vi "Begin.vi"() -> (0 "error out":errorcluster)   [LabVIEW 2013]
doc: "Called before other user functions, this VI is expected to open initial I/O refnums, load in file data, and do all program initialization. Notice that the <B>error out</B> terminal is simply used for data flow. Wiring it to other structures or subVIs ensures that this VI runs first."
uses:
  <vilib>/Rock Robotics/WPI/Camera/WPI_CameraImageSize.ctl
  <vilib>/Rock Robotics/SystemInterfaces/DIO/FPGA_DIOPWMChannel.ctl
  <vilib>/Rock Robotics/WPI/DriverStation/WPI_DriverStationRobotMode2.ctl
  <vilib>/Rock Robotics/WPI/Joystick/WPI_JoystickDeviceEnum.ctl
  <vilib>/Rock Robotics/SystemInterfaces/DIO/FPGA_DIOChannel.ctl
  <vilib>/Rock Robotics/WPI/Camera/WPI_CameraWhite Balance Values.ctl
  <vilib>/Rock Robotics/WPI/Camera/WPI_CameraExposure Values.ctl
  <vilib>/Rock Robotics/WPI/Camera/WPI_CameraFrameRate.ctl
  <vilib>/Rock Robotics/SystemInterfaces/Typedef/FPGA_TypedefSolenoidModule.ctl
  <vilib>/Rock Robotics/WPI/Solenoid/WPI_SolenoidChannel.ctl
  <vilib>/Rock Robotics/SystemInterfaces/Typedef/FPGA_TypedefDigitalModule.ctl
  <vilib>/Rock Robotics/SystemInterfaces/DIO/FPGA_DIORelayChannel.ctl
  <vilib>/Rock Robotics/SystemInterfaces/Typedef/FPGA_TypedefAnalogModule.ctl
  <vilib>/Rock Robotics/SystemInterfaces/AI/FPGA_AIChannel.ctl
  <vilib>/Rock Robotics/WPI/Encoder/WPI_EncoderType.ctl
  <vilib>/Rock Robotics/WPI/Relay/WPI_RelayDirection.ctl
  <vilib>/Rock Robotics/WPI/RobotDrive/WPI_RobotDriveOpen2MotorWithTalon.vi
  Robot Global Data.vi
  <vilib>/Rock Robotics/WPI/MotorControl/WPI_MotorControlOpen Talon.vi
  <vilib>/Rock Robotics/WPI/Counter/WPI_CounterDigitalInputToDigitalSource.vi
  <vilib>/Rock Robotics/WPI/Solenoid/WPI_SolenoidOpenDouble.vi
  <vilib>/Rock Robotics/WPI/Compressor/WPI_CompressorGetSetRefNum.vi
panel:
  in  "Image Size 2":T1=enum."160x120"
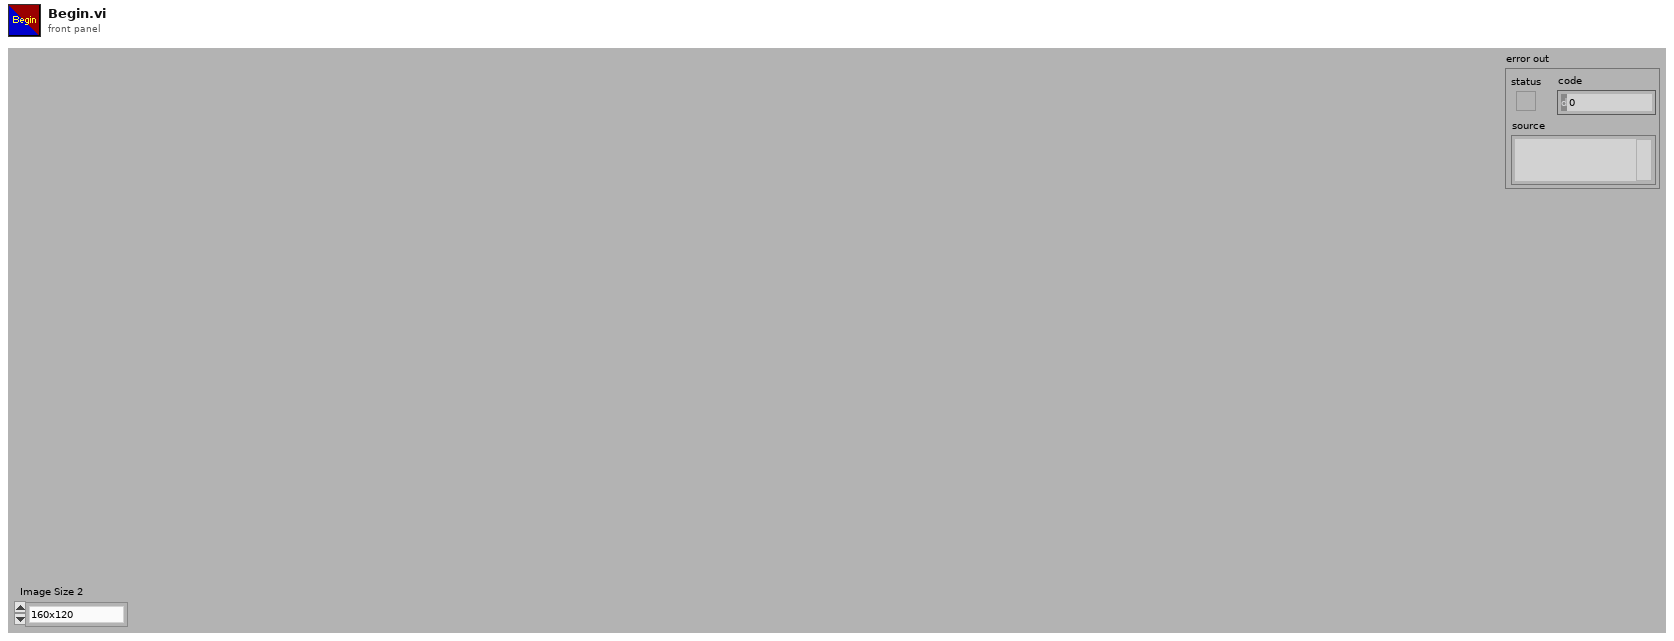
[diagram p1: front panel]
types:
  T1 = typedef "WPI_CameraImageSize.ctl" = enum16{"640x480", "320x240", "160x120"}
  T2 = typedef "WPI_JoystickDeviceEnum.ctl" = enum16{"USB 1", "USB 2", "USB 3", "USB 4", "Kinect 1", "Kinect 2"}
  T3 = typedef "WPI_RelayDirection.ctl" = enum16{"Both directions", "Forward only", "Reverse only"}
  T4 = typedef "FPGA_DIORelayChannel.ctl" = enum8{"Relay 1", "Relay 2", "Relay 3", "Relay 4", "Relay 5", "Relay 6", "Relay 7", "Relay 8", "Invalid"}
  T5 = typedef "FPGA_TypedefDigitalModule.ctl" = enum16{"Digital Module 1", "Digital Module 2"}
  T6 = typedef "FPGA_DIOChannel.ctl" = enum8{"DIO 1", "DIO 2", "DIO 3", "DIO 4", "DIO 5", "DIO 6", "DIO 7", "DIO 8", "DIO 9", "DIO 10", "DIO 11", "DIO 12", "DIO 13", "DIO 14", "Invalid"}
  T7 = typedef "WPI_EncoderType.ctl" = enum16{"1x", "2x", "4x"}
  T8 = typedef "FPGA_AIChannel.ctl" = enum8{"AI 1", "AI 2", "AI 3", "AI 4", "AI 5", "AI 6", "AI 7", "AI 8", "Invalid"}
  T9 = typedef "FPGA_TypedefAnalogModule.ctl" = enum16{"Analog Module 1", "Analog Module 2"}
  T10 = typedef "WPI_SolenoidChannel.ctl" = enum8{"Solenoid 1", "Solenoid 2", "Solenoid 3", "Solenoid 4", "Solenoid 5", "Solenoid 6", "Solenoid 7", "Solenoid 8", "Invalid"}
  T11 = typedef "FPGA_TypedefSolenoidModule.ctl" = enum16{"Solenoid Module 1", "Solenoid Module 2"}
  T12 = typedef "FPGA_DIOPWMChannel.ctl" = enum8{"PWM 1", "PWM 2", "PWM 3", "PWM 4", "PWM 5", "PWM 6", "PWM 7", "PWM 8", "PWM 9", "PWM 10", "Invalid"}
  T13 = typedef "WPI_CameraFrameRate.ctl" = u32
  T14 = typedef "WPI_CameraExposure Values.ctl" = enum16{"Auto", "Flicker-free 50 Hz", "Flicker-free 60 Hz", "Hold current"}
  T15 = typedef "WPI_CameraWhite Balance Values.ctl" = enum16{"Auto", "Fixed indoor", "Fixed outdoor 1", "Fixed outdoor 2", "Fixed fluorescent 1", "Fixed fluorescent 2", "Hold current"}
  T16 = typedef "WPI_DriverStationRobotMode2.ctl" = enum16{"Autonomous Disabled", "Autonomous Enabled", "Teleop Disabled", "Teleop Enabled", "Timeout", "Finish", "Test Disabled", "Test Enabled"}
  T17 = typedef "WPI_DigitalInputDevRef.ctl" = cluster{"DevStatus":errorcluster, "DIO Channel":T6, "Digital Module":T5}
  T18 = typedef "FPGA_CounterEncoderSourceConvertionLVSourceType.ctl" = cluster{"DevStatus":errorcluster, "AnalogTriggerMode?":bool, "DigitalMode":cluster{"Digital Module":T5, "DIO Channel":T19}, "AnalogTriggerMode":cluster{"AnalogTriggerIndex":T20, "OutputType":T21}}
  T19 = typedef "FPGA_DIODigitalSourceChannel.ctl" = enum8{"DIO 1", "DIO 2", "DIO 3", "DIO 4", "DIO 5", "DIO 6", "DIO 7", "DIO 8", "DIO 9", "DIO 10", "DIO 11", "DIO 12", "DIO 13", "DIO 14", "Disabled"}
  T20 = typedef "FPGA_AnalogTriggerIndex.ctl" = enum8{"Trig 0", "Trig 1", "Trig 2", "Trig 3", "Trig 4", "Trig 5", "Trig 6", "Trig 7", "Invalid"}
  T21 = typedef "FPGA_AnalogTriggerOutType.ctl" = enum16{"InWindow", "TriggerState", "Rising", "Falling"}
  T22 = typedef "WPI_EncoderDevRef.ctl" = cluster{"DevStatus":errorcluster, "EncoderIndex":T23, "CounterIndex":T24, "DistancePerCount":dbl, "Decoding Type":T7}
  T23 = typedef "FPGA_EncoderIdx.ctl" = enum8{"Enc 0", "Enc 1", "Enc 2", "Enc 3", "Invalid"}
  T24 = typedef "FPGA_CounterCtrSystemIndex.ctl" = enum8{"Ctr 0", "Ctr 1", "Ctr 2", "Ctr 3", "Ctr 4", "Ctr 5", "Ctr 6", "Ctr 7", "Invalid"}
  T25 = typedef "WPI_JoystickDevRef.ctl" = cluster{"Device":T2}
  T26 = typedef "WPI_CompressorDevRef.ctl" = cluster{"DevStatus":errorcluster, "DigitalInputDevRef":T17, "RelayDevRef":T27}
  T27 = typedef "WPI_RelayDevRef.ctl" = cluster{"DevStatus":errorcluster, "Relay Channel":T4, "Digital Module":T5, "Relay Direction":T3}
  T28 = typedef "WPI_RobotDriveDevRef.ctl" = cluster{"DevStatus":errorcluster, "Motors[]":T29[], "Square Inputs":bool, "Max Output":dbl, "Isochronous":bool}
  T29 = typedef "WPI_MotorControlDeviceRef.ctl" = cluster{"DeviceStatus":errorcluster, "Type":enum16{"PWM", "CAN"}, "PWM":cluster{"Digital Module":T5, "PWM Channel":T12, "DeadBand":T30}, "CAN":cluster{"Device Number":u8, "Control Mode":T31, "Semaphore":T32, "Max Vout":dbl}, "Invert":bool, "TransformRef":T33, "InvTransformRef":T33}
  T30 = typedef "WPI_PWMDeadband.ctl" = cluster{"Name":string, "maxPositivePwm":i32, "minPositivePwm":i32, "centerPwm":i32, "maxNegativePwm":i32, "minNegativePwm":i32, "angularRange":u16}
  T31 = typedef "WPI_CANJaguar_ControlMode.ctl" = enum8{"Percent VBus", "Current", "Speed", "Position", "Voltage"}
  T32 = typedef "Semaphore RefNum" = refnum<k1>
  T33 = typedef "WPI_PWMTransform_ConPane.ctl" = refnum<vi>
  T34 = typedef "WPI_SolenoidDevRef.ctl" = cluster{"DevStatus":errorcluster, "Solenoid Module":T11, "Forward Solenoid Channel":T10, "Reverse Solenoid Channel":T10}
  T35 = typedef "WPI_CameraDevRef.ctl" = cluster{"Camera Address":string, "CameraStatus":errorcluster, "Acquire Image Notifier":refnum<notifier>}
  T36 = typedef "WPI_ServoDeviceRef.ctl" = cluster{"DeviceStatus":errorcluster, "Digital Module":T5, "PWM Channel":T12, "DeadBand":T30}
  T37 = typedef "WPI_AnalogChannelDevRef.ctl" = cluster{"DevStatus":errorcluster, "Analog Module":T9, "Analog Channel":T8}
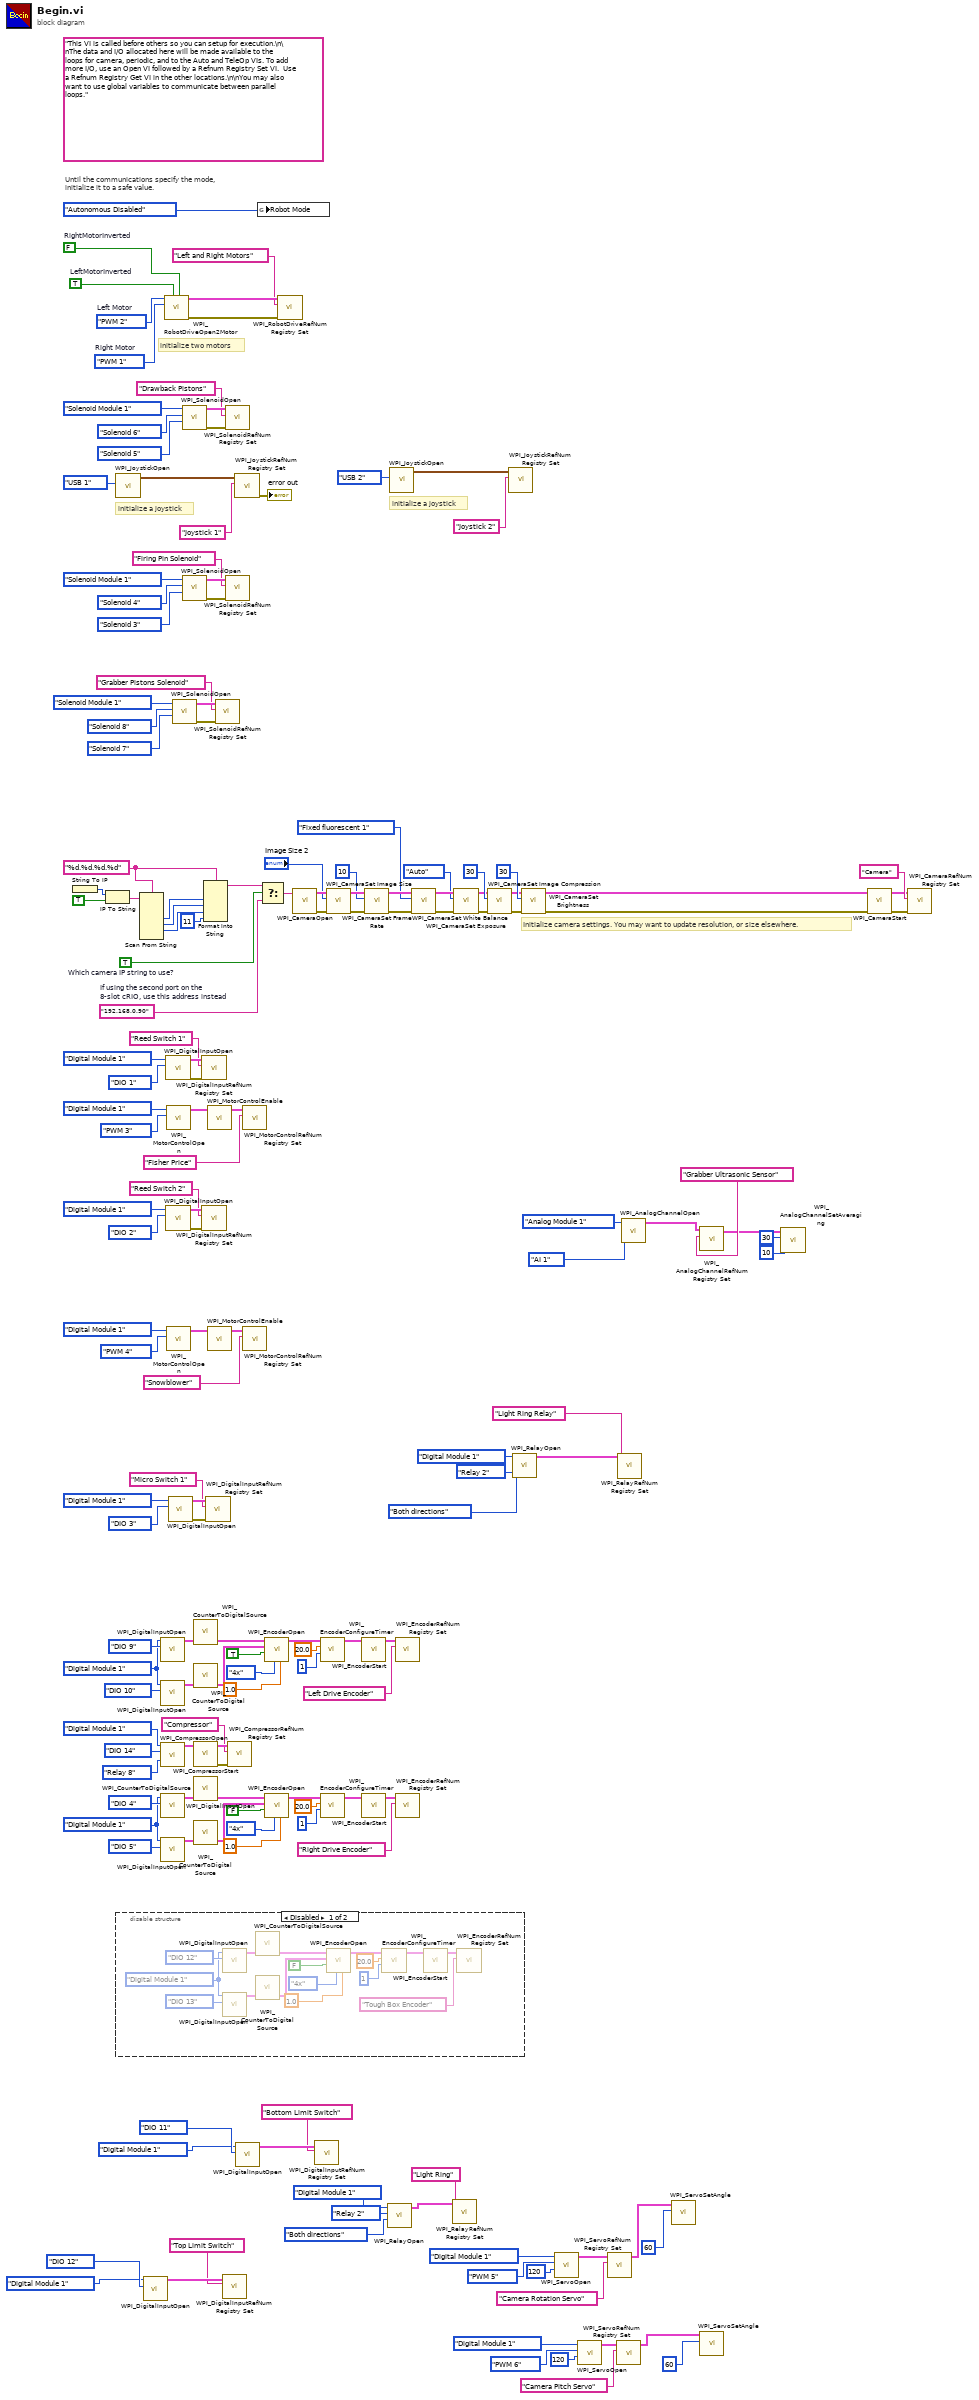
[diagram p0: block diagram]
diagram:
  w25 = FPGA_TypedefDigitalModule."Digital Module 1" ("DIO Module")
  w108 = TRUE  # Which camera IP string to use?
  w112 = "%d.%d.%d.%d" ("format string")
  w109 = "192.168.0.90"  # If using the second port on the 8-slot cRIO, use this address instead
  w141 = FPGA_TypedefDigitalModule."Digital Module 1" ("DIO Module")
  (unwired) "This VI is called before others so you can setup for execution.\n\nThe data and I/O allocated here will be made available to the loops for camera, periodic, and to the Auto and TeleOp VIs. To add more I/O, use an Open VI followed by a Refnum Registry Set VI.  Use a Refnum Registry Get VI in the other locations.\n\nYou may also want to use global variables to communicate between parallel loops."
  w165 = FPGA_DIOPWMChannel."PWM 1"  # Right Motor
  w166 = FPGA_DIOPWMChannel."PWM 2"  # Left Motor
  w170 = TRUE  # LeftMotorInverted
  w171 = FALSE  # RightMotorInverted
  # "initialize a joystick"
  # "Initialize camera settings. You may want to update resolution, or size elsewhere."
  # "initialize a joystick"
  # "Until the communications specify the mode,\ninitialize it to a safe value."
  # "initialize two motors"
  n1 = String To IP() -> (0:w119:u32)  [unwired: 1 in]
  n2 = IP To String(1:TRUE ("dot notation? (F)"), 2:w119) -> (0:w117:string)
  n3 = disable-structure shown="Disabled" {
    frame Disabled {
      w174 = FPGA_TypedefDigitalModule."Digital Module 1" ("DIO Module")
      n4 = call <vilib>:"WPI_DigitalInputOpen.vi"("DIO Channel"=FPGA_DIOChannel."DIO 12" ("A Channel"), "Digital Module (Module 1)"=w174) -> ("DigitalInputDevRef"=w185:T17)  [unwired: 1 in, 8 out]
      n5 = call <vilib>:"WPI_DigitalInputOpen.vi"("DIO Channel"=FPGA_DIOChannel."DIO 13" ("B Channel"), "Digital Module (Module 1)"=w174) -> ("DigitalInputDevRef"=w186:T17)  [unwired: 1 in, 8 out]
      n6 = call-poly <vilib>:"WPI_CounterToDigitalSource.vi"("DigitalInputDevRef"=w185) -> ("Digital Source"=w184:T18)  [unwired: 6 out]
      n7 = call-poly <vilib>:"WPI_CounterToDigitalSource.vi"("DigitalInputDevRef"=w186) -> ("Digital Source"=w187:T18)  [unwired: 6 out]
      n8 = call <vilib>:"WPI_EncoderOpen.vi"("DistancePerCount"=1.0, "Decoding Type"=WPI_EncoderType."4x", "Invert Direction (False)"=FALSE ("Invert Direction"), "BSource"=w187, "ASource"=w184) -> ("EncoderDevRef"=w177:T22)  [unwired: 3 in, 3 out]
      n9 = call <vilib>:"WPI_EncoderConfigureTimer.vi"("Number Samples to Average"=u8 1, "Minimum Rate"=20.0, "EncoderDevRef"=w177) -> ("EncoderDevRef"=w178:T22)  [unwired: 1 in, 7 out]
      n10 = call <vilib>:"WPI_EncoderStart.vi"("EncoderDevRef"=w178) -> ("EncoderDevRef"=w173:T22)  [unwired: 1 in, 9 out]
      n11 = call <vilib>:"WPI_EncoderRefNum Registry Set.vi"("refnum name"="Tough Box Encoder", "EncoderDevRef"=w173) -> ()  [unwired: 8 in, 2 out]
    }
    frame Enabled {
    }
  }
  n12 = call <vilib>:"WPI_JoystickOpen.vi"("JoystickDevice"=WPI_JoystickDeviceEnum."USB 1") -> ("JoystickDevRef"=w162:T25)  [unwired: 10 in]
  n13 = Scan From String(format string=w112, input string=w117) -> (output 1=w116:i32, output 2=w115:i32, output 3=w114:i32)  [unwired: 7 in, 3 out]
  n14 = call <vilib>:"WPI_DigitalInputOpen.vi"("DIO Channel"=FPGA_DIOChannel."DIO 12" ("A Channel"), "Digital Module (Module 1)"=FPGA_TypedefDigitalModule."Digital Module 1" ("DIO Module")) -> ("DigitalInputDevRef"=w40:T17)  [unwired: 8 in, 1 out]
  n15 = call <vilib>:"WPI_DigitalInputOpen.vi"("DIO Channel"=FPGA_DIOChannel."DIO 9" ("A Channel"), "Digital Module (Module 1)"=w25) -> ("DigitalInputDevRef"=w36:T17)  [unwired: 1 in, 8 out]
  n16 = call <vilib>:"WPI_DigitalInputOpen.vi"("DIO Channel"=FPGA_DIOChannel."DIO 10" ("B Channel"), "Digital Module (Module 1)"=w25) -> ("DigitalInputDevRef"=w37:T17)  [unwired: 1 in, 8 out]
  n17 = call <vilib>:"WPI_CompressorOpen.vi"("Pressure Switch Digital Module (Module 1)"=FPGA_TypedefDigitalModule."Digital Module 1" ("Switch and Relay Module"), "Pressure Switch DIO Channel"=FPGA_DIOChannel."DIO 14" ("Pressure Switch Channel"), "Relay Channel"=FPGA_DIORelayChannel."Relay 8" ("RelayChannel")) -> ("CompressorDevRef"=w96:T26)  [unwired: 2 in, 10 out]
  n18 = call <vilib>:"WPI_DigitalInputOpen.vi"("DIO Channel"=FPGA_DIOChannel."DIO 4" ("A Channel"), "Digital Module (Module 1)"=w141) -> ("DigitalInputDevRef"=w152:T17)  [unwired: 1 in, 8 out]
  n19 = call <vilib>:"WPI_DigitalInputOpen.vi"("DIO Channel"=FPGA_DIOChannel."DIO 5" ("B Channel"), "Digital Module (Module 1)"=w141) -> ("DigitalInputDevRef"=w153:T17)  [unwired: 1 in, 8 out]
  n20 = call-poly <vilib>:"WPI_RobotDriveOpen2Motor.vi"("Right Motor Inverted"=w171, "Left Motor Inverted"=w170, "Right Motor"=w165, "Left Motor"=w166) -> ("error out"=w167:errorcluster, "RobotDriveDevRef"=w169:T28)  [unwired: 1 in, 5 out]
  n21 = call <vilib>:"WPI_DigitalInputOpen.vi"("DIO Channel"=FPGA_DIOChannel."DIO 1" ("Limit Switch Channel"), "Digital Module (Module 1)"=FPGA_TypedefDigitalModule."Digital Module 1" ("Switch and Relay Module")) -> ("error out"=w95:errorcluster, "DigitalInputDevRef"=w94:T17)  [unwired: 1 in, 7 out]
  n22 = call <vilib>:"WPI_DigitalInputOpen.vi"("DIO Channel"=FPGA_DIOChannel."DIO 2" ("Limit Switch Channel"), "Digital Module (Module 1)"=FPGA_TypedefDigitalModule."Digital Module 1" ("Switch and Relay Module")) -> ("error out"=w77:errorcluster, "DigitalInputDevRef"=w76:T17)  [unwired: 1 in, 7 out]
  n23 = call-poly <vilib>:"WPI_MotorControlOpen.vi"("PWM Channel"=FPGA_DIOPWMChannel."PWM 3" ("Left Motor"), "Digital Module (Module 1)"=enum16{"Digital Module 1"}."Digital Module 1") -> ("MotorControlDeviceRef"=w73:T29)  [unwired: 8 in, 1 out]
  n24 = call-poly <vilib>:"WPI_MotorControlOpen.vi"("PWM Channel"=FPGA_DIOPWMChannel."PWM 4" ("Left Motor"), "Digital Module (Module 1)"=enum16{"Digital Module 1"}."Digital Module 1") -> ("MotorControlDeviceRef"=w71:T29)  [unwired: 8 in, 1 out]
  n25 = call <vilib>:"WPI_DigitalInputOpen.vi"("DIO Channel"=FPGA_DIOChannel."DIO 3", "Digital Module (Module 1)"=FPGA_TypedefDigitalModule."Digital Module 1") -> ("error out"=w19:errorcluster, "DigitalInputDevRef"=w20:T17)  [unwired: 1 in, 7 out]
  n26 = call-poly <vilib>:"WPI_SolenoidOpen.vi"("Reverse Solenoid Channel"=WPI_SolenoidChannel."Solenoid 7" ("Extend Solenoid Channel"), "Forward Solenoid Channel"=WPI_SolenoidChannel."Solenoid 8" ("Retract Solenoid Channel"), "Solenoid Module (Module 1)"=FPGA_TypedefSolenoidModule."Solenoid Module 1" ("Solenoid Module")) -> ("error out"=w52:errorcluster, "SolenoidDevRef"=w51:T34)  [unwired: 1 in, 6 out]
  n27 = call-poly <vilib>:"WPI_SolenoidOpen.vi"("Reverse Solenoid Channel"=WPI_SolenoidChannel."Solenoid 5" ("Extend Solenoid Channel"), "Forward Solenoid Channel"=WPI_SolenoidChannel."Solenoid 6" ("Retract Solenoid Channel"), "Solenoid Module (Module 1)"=FPGA_TypedefSolenoidModule."Solenoid Module 1" ("Solenoid Module")) -> ("error out"=w92:errorcluster, "SolenoidDevRef"=w91:T34)  [unwired: 1 in, 6 out]
  n28 = call-poly <vilib>:"WPI_SolenoidOpen.vi"("Reverse Solenoid Channel"=WPI_SolenoidChannel."Solenoid 3" ("Extend Solenoid Channel"), "Forward Solenoid Channel"=WPI_SolenoidChannel."Solenoid 4" ("Retract Solenoid Channel"), "Solenoid Module (Module 1)"=FPGA_TypedefSolenoidModule."Solenoid Module 1" ("Solenoid Module")) -> ("error out"=w83:errorcluster, "SolenoidDevRef"=w82:T34)  [unwired: 1 in, 6 out]
  n29 = call-poly <vilib>:"WPI_CounterToDigitalSource.vi"("DigitalInputDevRef"=w36) -> ("Digital Source"=w35:T18)  [unwired: 6 out]
  n30 = call-poly <vilib>:"WPI_CounterToDigitalSource.vi"("DigitalInputDevRef"=w37) -> ("Digital Source"=w38:T18)  [unwired: 6 out]
  n31 = call <vilib>:"WPI_CompressorStart.vi"("CompressorDevRef"=w96) -> ("error out"=w89:errorcluster, "CompressorDevRef"=w88:T26)  [unwired: 1 in, 8 out]
  n32 = call-poly <vilib>:"WPI_CounterToDigitalSource.vi"("DigitalInputDevRef"=w152) -> ("Digital Source"=w151:T18)  [unwired: 6 out]
  n33 = call-poly <vilib>:"WPI_CounterToDigitalSource.vi"("DigitalInputDevRef"=w153) -> ("Digital Source"=w154:T18)  [unwired: 6 out]
  n34 = call <vilib>:"WPI_DigitalInputRefNum Registry Set.vi"("error in (no error)"=w95, "refnum name"="Reed Switch 1", "DigitalInputDevRef"=w94) -> ()  [unwired: 7 in, 2 out]
  n35 = call <vilib>:"WPI_DigitalInputRefNum Registry Set.vi"("error in (no error)"=w77, "refnum name"="Reed Switch 2", "DigitalInputDevRef"=w76) -> ()  [unwired: 7 in, 2 out]
  n36 = Format Into String(format string=w112, w116, w115, w114, 11 ("Compression")) -> (resulting string=w110:string)  [unwired: 2 in, 1 out]
  n37 = call <vilib>:"WPI_DigitalInputRefNum Registry Set.vi"("error in (no error)"=w19, "refnum name"="Micro Switch 1", "DigitalInputDevRef"=w20) -> ()  [unwired: 7 in, 2 out]
  n38 = call <vilib>:"WPI_MotorControlEnable.vi"("CAN Jaguar Ref"=w73) -> ("CAN Jaguar Ref Out"=w72:T29)  [unwired: 9 in, 1 out]
  n39 = call <vilib>:"WPI_MotorControlEnable.vi"("CAN Jaguar Ref"=w71) -> ("CAN Jaguar Ref Out"=w70:T29)  [unwired: 9 in, 1 out]
  n40 = call <vilib>:"WPI_SolenoidRefNum Registry Set.vi"("error in (no error)"=w52, "refnum name"="Grabber Pistons Solenoid", "SolenoidDevRef"=w51) -> ()  [unwired: 7 in, 2 out]
  n41 = call <vilib>:"WPI_DigitalInputRefNum Registry Set.vi"("refnum name"="Top Limit Switch", "DigitalInputDevRef"=w40) -> ()  [unwired: 8 in, 2 out]
  n42 = call <vilib>:"WPI_SolenoidRefNum Registry Set.vi"("error in (no error)"=w92, "refnum name"="Drawback Pistons", "SolenoidDevRef"=w91) -> ()  [unwired: 7 in, 2 out]
  n43 = call <vilib>:"WPI_SolenoidRefNum Registry Set.vi"("error in (no error)"=w83, "refnum name"="Firing Pin Solenoid", "SolenoidDevRef"=w82) -> ()  [unwired: 7 in, 2 out]
  n44 = call <vilib>:"WPI_CompressorRefNum Registry Set.vi"("error in (no error)"=w89, "refnum name"="Compressor", "CompressorDevRef"=w88) -> ()  [unwired: 7 in, 2 out]
  n45 = call <vilib>:"WPI_JoystickRefNum Registry Set.vi"("refnum name"="Joystick 1", "JoystickDevRef"=w162) -> ("error out"=→"error out":errorcluster)  [unwired: 8 in, 1 out]
  n46 = call <vilib>:"WPI_DigitalInputOpen.vi"("DIO Channel"=FPGA_DIOChannel."DIO 11" ("A Channel"), "Digital Module (Module 1)"=FPGA_TypedefDigitalModule."Digital Module 1" ("DIO Module")) -> ("DigitalInputDevRef"=w67:T17)  [unwired: 8 in, 1 out]
  n47 = call <vilib>:"WPI_MotorControlRefNum Registry Set.vi"("refnum name"="Fisher Price", "MotorControlDevRef"=w72) -> ()  [unwired: 8 in, 2 out]
  n48 = call <vilib>:"WPI_MotorControlRefNum Registry Set.vi"("refnum name"="Snowblower", "MotorControlDevRef"=w70) -> ()  [unwired: 8 in, 2 out]
  n49 = global write "Robot Global Data.vi" "Robot Mode"(WPI_DriverStationRobotMode2."Autonomous Disabled" ("Robot Mode")) -> ()
  n50 = Select(t=w110, s=w108, f=w109) -> (s? t:f=w111:string)
  n51 = call <vilib>:"WPI_EncoderOpen.vi"("DistancePerCount"=1.0, "Decoding Type"=WPI_EncoderType."4x", "Invert Direction (False)"=TRUE ("Invert Direction"), "BSource"=w38, "ASource"=w35) -> ("EncoderDevRef"=w28:T22)  [unwired: 3 in, 3 out]
  n52 = call <vilib>:"WPI_EncoderOpen.vi"("DistancePerCount"=1.0, "Decoding Type"=WPI_EncoderType."4x", "Invert Direction (False)"=FALSE ("Invert Direction"), "BSource"=w154, "ASource"=w151) -> ("EncoderDevRef"=w144:T22)  [unwired: 3 in, 3 out]
  n53 = call <vilib>:"WPI_RobotDriveRefNum Registry Set.vi"("error in (no error)"=w167, "refnum name"="Left and Right Motors", "RobotDriveDevRef"=w169) -> ()  [unwired: 9 out]
  n54 = call <vilib>:"WPI_CameraOpen.vi"("Camera Address"=w111) -> ("error out"=w129:errorcluster, "CameraDevRef"=w130:T35)  [unwired: 1 in, 8 out]
  n55 = call <vilib>:"WPI_DigitalInputRefNum Registry Set.vi"("refnum name"="Bottom Limit Switch", "DigitalInputDevRef"=w67) -> ()  [unwired: 8 in, 2 out]
  n56 = call <vilib>:"WPI_EncoderConfigureTimer.vi"("Number Samples to Average"=u8 1, "Minimum Rate"=20.0, "EncoderDevRef"=w28) -> ("EncoderDevRef"=w29:T22)  [unwired: 1 in, 7 out]
  n57 = call <vilib>:"WPI_EncoderConfigureTimer.vi"("Number Samples to Average"=u8 1, "Minimum Rate"=20.0, "EncoderDevRef"=w144) -> ("EncoderDevRef"=w145:T22)  [unwired: 1 in, 7 out]
  n58 = call <vilib>:"WPI_CameraSet Image Size.vi"("error in (no error)"=w129, "Image Size"="Image Size 2", "CameraDevRef"=w130) -> ("error out"=w128:errorcluster, "CameraDevRef Out"=w131:T35)  [unwired: 7 out]
  n59 = call <vilib>:"WPI_EncoderStart.vi"("EncoderDevRef"=w29) -> ("EncoderDevRef"=w24:T22)  [unwired: 1 in, 9 out]
  n60 = call <vilib>:"WPI_EncoderStart.vi"("EncoderDevRef"=w145) -> ("EncoderDevRef"=w140:T22)  [unwired: 1 in, 9 out]
  n61 = call <vilib>:"WPI_CameraSet Frame Rate.vi"("error in (no error)"=w128, "Frame Rate (fps)"=T13 10, "CameraDevRef"=w131) -> ("error out"=w127:errorcluster, "CameraDevRef Out"=w133:T35)  [unwired: 7 out]
  n62 = call <vilib>:"WPI_RelayOpen.vi"("Relay Direction"=WPI_RelayDirection."Both directions", "Relay Channel"=FPGA_DIORelayChannel."Relay 2", "Digital Module (Module 1)"=FPGA_TypedefDigitalModule."Digital Module 1") -> ("RelayDevRef"=w9:T27)  [unwired: 7 in, 1 out]
  n63 = call <vilib>:"WPI_JoystickOpen.vi"("JoystickDevice"=WPI_JoystickDeviceEnum."USB 2") -> ("JoystickDevRef"=w2:T25)  [unwired: 10 in]
  n64 = call <vilib>:"WPI_EncoderRefNum Registry Set.vi"("refnum name"="Left Drive Encoder", "EncoderDevRef"=w24) -> ()  [unwired: 8 in, 2 out]
  n65 = call <vilib>:"WPI_EncoderRefNum Registry Set.vi"("refnum name"="Right Drive Encoder", "EncoderDevRef"=w140) -> ()  [unwired: 8 in, 2 out]
  n66 = call <vilib>:"WPI_CameraSet White Balance.vi"("error in (no error)"=w127, "White Balance"=WPI_CameraWhite_Balance_Values."Fixed fluorescent 1", "CameraDevRef"=w133) -> ("error out"=w126:errorcluster, "CameraDevRef Out"=w132:T35)  [unwired: 7 out]
  n67 = call <vilib>:"WPI_RelayRefNum Registry Set.vi"("refnum name"="Light Ring", "RelayDevRef"=w9) -> ()  [unwired: 8 in, 2 out]
  n68 = call <vilib>:"WPI_CameraSet Exposure.vi"("error in (no error)"=w126, "Exposure"=WPI_CameraExposure_Values."Auto", "CameraDevRef"=w132) -> ("error out"=w125:errorcluster, "CameraDevRef Out"=w135:T35)  [unwired: 7 out]
  n69 = call <vilib>:"WPI_CameraSet Image Compression.vi"("error in (no error)"=w125, "Compression"=30, "CameraDevRef"=w135) -> ("error out"=w124:errorcluster, "CameraDevRef Out"=w134:T35)  [unwired: 7 out]
  n70 = call <vilib>:"WPI_JoystickRefNum Registry Set.vi"("refnum name"="Joystick 2", "JoystickDevRef"=w2) -> ()  [unwired: 8 in, 2 out]
  n71 = call <vilib>:"WPI_RelayOpen.vi"("Relay Direction"=WPI_RelayDirection."Both directions", "Relay Channel"=FPGA_DIORelayChannel."Relay 2", "Digital Module (Module 1)"=FPGA_TypedefDigitalModule."Digital Module 1") -> ("RelayDevRef"=w14:T27)  [unwired: 7 in, 1 out]
  n72 = call <vilib>:"WPI_CameraSet Brightness.vi"("error in (no error)"=w124, "Brightness"=30, "CameraDevRef"=w134) -> ("error out"=w107:errorcluster, "CameraDevRef Out"=w106:T35)  [unwired: 7 out]
  n73 = call <vilib>:"WPI_ServoOpen.vi"("Angular Range"=u16 120, "PWM Channel"=FPGA_DIOPWMChannel."PWM 5", "Digital Module (Module 1)"=FPGA_TypedefDigitalModule."Digital Module 1") -> ("ServoDeviceRef"=w58:T36)  [unwired: 7 in, 1 out]
  n74 = call <vilib>:"WPI_ServoOpen.vi"("Angular Range"=u16 120, "PWM Channel"=FPGA_DIOPWMChannel."PWM 6", "Digital Module (Module 1)"=FPGA_TypedefDigitalModule."Digital Module 1") -> ("ServoDeviceRef"=w59:T36)  [unwired: 7 in, 1 out]
  n75 = call <vilib>:"WPI_ServoRefNum Registry Set.vi"("refnum name"="Camera Rotation Servo", "ServoDeviceRef"=w58) -> ("ServoDeviceRef"=w7:T36)  [unwired: 8 in, 1 out]
  n76 = call <vilib>:"WPI_ServoRefNum Registry Set.vi"("refnum name"="Camera Pitch Servo", "ServoDeviceRef"=w59) -> ("ServoDeviceRef"=w5:T36)  [unwired: 8 in, 1 out]
  n77 = call <vilib>:"WPI_RelayRefNum Registry Set.vi"("refnum name"="Light Ring Relay", "RelayDevRef"=w14) -> ()  [unwired: 8 in, 2 out]
  n78 = call <vilib>:"WPI_AnalogChannelOpen.vi"("Analog Channel"=FPGA_AIChannel."AI 1", "Analog Module (Module 1)"=FPGA_TypedefAnalogModule."Analog Module 1") -> ("AIDeviceRef"=w47:T37)  [unwired: 8 in, 1 out]
  n79 = call <vilib>:"WPI_ServoSetAngle.vi"("Angle"=60, "ServoDeviceRef"=w7) -> ()  [unwired: 8 in, 2 out]
  n80 = call <vilib>:"WPI_AnalogChannelRefNum Registry Set.vi"("refnum name"="Grabber Ultrasonic Sensor", "AIDeviceRef"=w47) -> ("AIDeviceRef"=w45:T37)  [unwired: 8 in, 1 out]
  n81 = call <vilib>:"WPI_ServoSetAngle.vi"("Angle"=60, "ServoDeviceRef"=w5) -> ()  [unwired: 8 in, 2 out]
  n82 = call <vilib>:"WPI_AnalogChannelSetAveraging.vi"("OversampleBits"=u8 10, "AverageBits"=u8 30, "AIDeviceRef"=w45) -> ()  [unwired: 7 in, 2 out]
  n83 = call <vilib>:"WPI_CameraStart.vi"("error in (no error)"=w107, "CameraDevRef"=w106) -> ("error out"=w105:errorcluster, "CameraDevRef Out"=w104:T35)  [unwired: 8 in]
  n84 = call <vilib>:"WPI_CameraRefNum Registry Set.vi"("error in (no error)"=w105, "refnum name"="Camera", "CameraDevRef"=w104) -> ()  [unwired: 9 out]
